vi "AlazarFFTBackgroundSubtractionGetRecordS16.vi"(4 "error in (no error)":errorcluster, 5 "Background Record In":i16[](array[numeric]), 7 "DSP Handle":u64) -> (0 "error out":errorcluster, 1 "Return Code":u32, 2 "Background Record Out":i16[](array[numeric]), 3 "DSP Handle":u64)   [LabVIEW 2018]
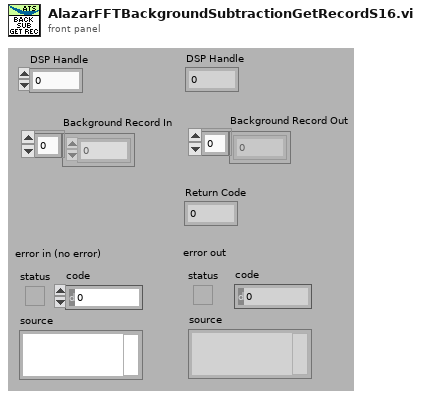
[diagram p1: front panel]
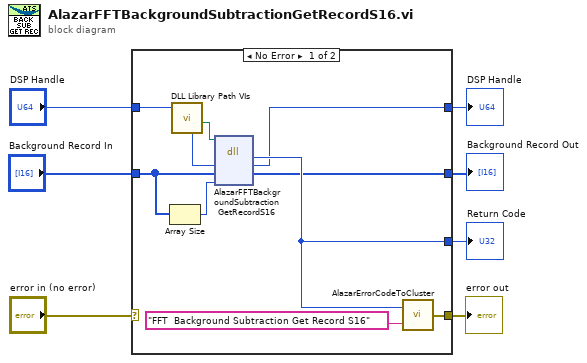
[diagram p0: block diagram]
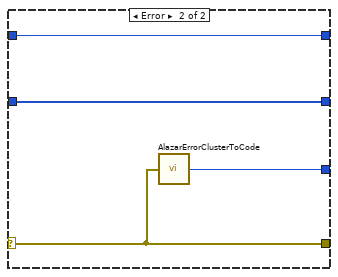
[diagram p2: hidden frame]
diagram:
  n1 = case shown="No Error" "error in (no error)" {
    selector: "error in (no error)" -> [_ w20]
    tunnel: [w13 w20] -> w6
    tunnel: [w15 w19] -> w2
    tunnel: "DSP Handle" -> [w16 w18]
    tunnel: [w12 w18] -> w4
    tunnel: "Background Record In" -> [w11 w17]
    tunnel: [w9 w17] -> w1
    frame No Error {
      n2 = Array Size(array=w11) -> (size(s)=w10:i32)
      n3 = call "DLL Library Path VIs.vi"() -> ("Alazar"=w8:path)  [unwired: 9 in, 2 out]
      n4 = dll-call lib="C:/Project/SerialSectOCT - FFT GPU/SerialSectOCT/Labview Software/DLL/ATSApi.dll" fn="AlazarFFTBackgroundSubtractionGetRecordS16"(path in=w8, "dspHandle"=w16, "backgroundRecord"=w11, "size_samples"=w10) -> ("return type"=w15:u32, "dspHandle"=w12:u64, "backgroundRecord"=w9:i16[])  [unwired: 3 in, 2 out]
      n5 = call "AlazarErrorCodeToCluster.vi"("Message"="FFT  Background Subtraction Get Record S16", "Error Code"=w15) -> ("error out"=w13:errorcluster)
    }
    frame Error {
      n6 = call "AlazarErrorClusterToCode.vi"("error in (no error)"=w20) -> ("Error Code"=w19:u32)
    }
  }
  "DSP Handle" <- w4
  "error out" <- w6
  "Return Code" <- w2
  "Background Record Out" <- w1
